vi "DA_Single_Out.vi"() -> ()   [LabVIEW 2012]
uses:
  Usb_Daq_V52_Dll.dll
panel:
  in  "stop":bool
  in  "电压":dbl min=0.0 max=10.0
  in  "通道":i32=1 min=0 max=1
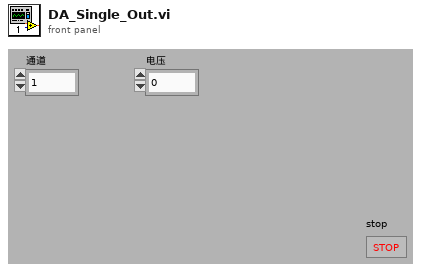
[diagram p1: front panel]
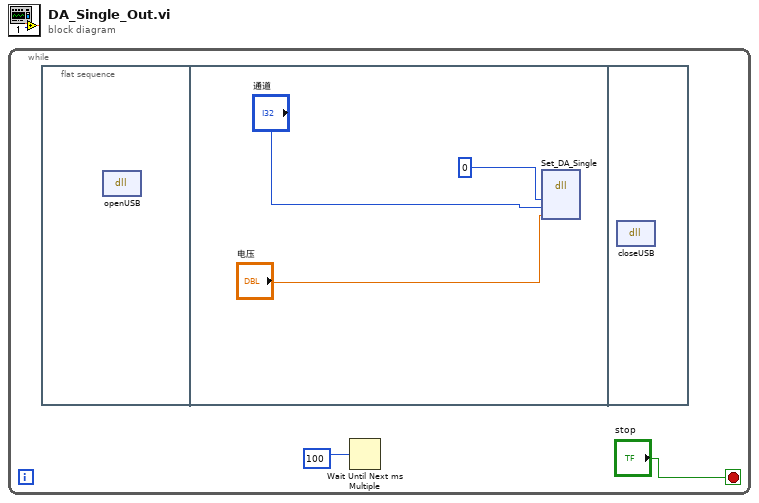
[diagram p0: block diagram]
diagram:
  n1 = while {
    stop <- "stop" stop-if-true
    n2 = flat-sequence {
      frame #0 {
        n3 = dll-call lib="PTH1labs Ebackup数据采集卡uSB!USB数据采集卡资料HKUSB6203例程labviewUsb_Daq_V52_Dll.dll" fn="openUSB"() -> ()  [unwired: 4 in, 2 out]
      }
      frame #1 {
        n4 = dll-call lib="PTH1labs Ebackup数据采集卡uSB!USB数据采集卡资料HKUSB6203例程labviewUsb_Daq_V52_Dll.dll" fn="Set_DA_Single"("dev"=0, "chan"="通道", "value"="电压") -> ()  [unwired: 7 in, 2 out]
      }
      frame #2 {
        n5 = dll-call lib="PTH1labs Ebackup数据采集卡uSB!USB数据采集卡资料HKUSB6203例程labviewUsb_Daq_V52_Dll.dll" fn="closeUSB"() -> ()  [unwired: 4 in, 2 out]
      }
    }
    n6 = Wait Until Next ms Multiple(millisecond multiple=100) -> ()  [unwired: 1 out]
  }
